vi "二级-力传-转换.vi"(11 "Waveform":dbl) -> (3 "Filtered x":dbl)   [LabVIEW 2020]
uses:
  <vilib>/ptbypt/NI_PtbyPt.lvlib
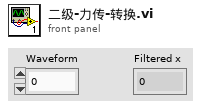
[diagram p1: front panel]
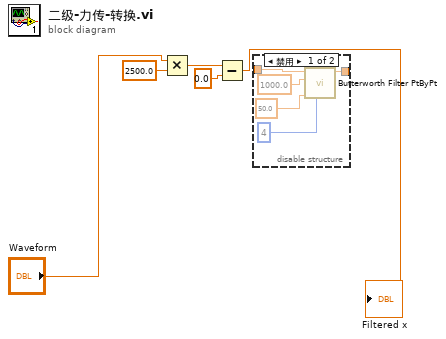
[diagram p0: block diagram]
diagram:
  n1 = Multiply(x="Waveform", y=2500.0) -> (x*y=w4:dbl)
  n2 = Subtract(x=w4, y=0.0) -> (x-y=→"Filtered x":dbl)
  n3 = disable-structure shown="禁用" {
    disable-tunnel: [w10 _] -> _
    disable-tunnel: _ -> [w9 _]
    frame Disabled {
      n4 = call <vilib>:"Butterworth Filter PtByPt.vi"("order"=4, "low cutoff freq: fl"=50.0, "sampling freq: fs"=1000.0, "x"=w9) -> ("Filtered x"=w10:dbl)  [unwired: 5 in, 1 out]
    }
    frame Enabled {
    }
  }
